vi "tt_offset.vi"() -> (0 "offset":dbl)   [LabVIEW 2013]
panel:
  out "x*y":dbl
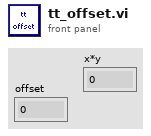
[diagram p1: front panel]
types:
  T1 = typedef "LVRectTypeDef.ctl" = cluster{"Left":i16, "Top":i16, "Right":i16, "Bottom":i16}
  T2 = cluster{"Xpixels":i32, "Vx-min ref":dbl, "Vx-max ref":dbl, "P":dbl, "Ypixels":i32, "Vy-min ref":dbl, "Vy-max ref":dbl, "srate":sgl, "sAOxy":i32, "timeout":dbl, "type":string, "date":string, "time":string, "Colormap":u16, "Drawing Mode":u16, "Scanning Mode":u16, "square pixels":bool, "square matrix":bool, "Xpixels Img":i32, "Vx-min Img":dbl, "VX-max Img":dbl, "Ypixels Img":i32, "Vy-min Img":dbl, "Vy-max Img ":dbl, "Angle Img":dbl, "autoshutter":bool, "finite":bool, "cont":bool, "wavdet":bool, "measpoints":i32, "avpp":i32, "bufferAO":i32, "bufferAI":i32, "CH1":bool, "CH2":bool, "X":bool, "Y":bool, "Ip":bool, "Vp":bool, "starttick":u32, "waveform":path, "Vx-ref":dbl, "Vy-ref":dbl, "refreshrate":dbl, "refreshbuffer":i32, "tt_cycles":i32, "motorref":refnum<k7>, "mirrorswitch":refnum<k7>, "sample mode":i32, "maxbufferAI":i32, "sampletreshold":dbl, "srateAODO":sgl, "bin":sgl, "Pel":sgl, "Angle draw":dbl, "srate Img":sgl, "ROIimg_plotbounds":T1}
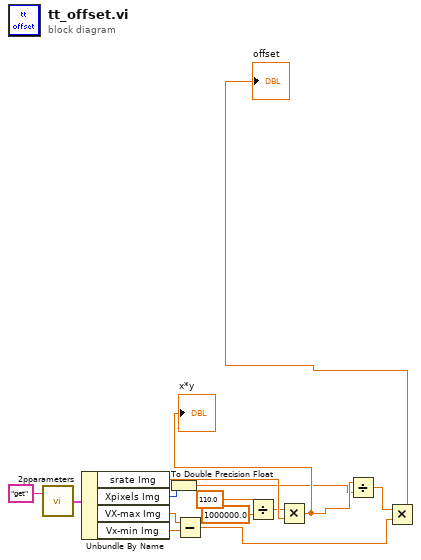
[diagram p0: block diagram]
diagram:
  n1 = call "2pparameters.vi"("command"="get") -> ("Params out"=w5:T2)  [unwired: 1 in]
  n2 = Unbundle By Name(w5) -> ("srate Img"=w9:sgl, "Xpixels Img"=w3:i32, "VX-max Img"=w10:dbl, "Vx-min Img"=w11:dbl)
  n3 = To Double Precision Float(number=w3) -> (double precision float=w1:dbl)
  n4 = Subtract(x=w10, y=w11) -> (x-y=w13:dbl)
  n5 = Divide(x=110.0, y=1000000.0) -> (x/y=w6:dbl)
  n6 = Multiply(x=w6, y=w9) -> (x*y=w2:dbl)
  "x*y" <- w2
  n7 = Divide(x=w2, y=w1) -> (x/y=w12:dbl)
  n8 = Multiply(x=w12, y=w13) -> (x*y=→"offset":dbl)
